vi "test launch & send msg to server.vi"() -> ()   [LabVIEW 2016, in "server.lvlib" / "server.lvclass"]
uses:
  server.lvclass
  C:/Program Files/National Instruments/LabVIEW 2016/vi.lib/ActorFramework/Actor/Actor.lvclass
  <vilib>/ActorFramework/Message Enqueuer/Message Enqueuer.lvclass/Message Enqueuer.ctl
  server Messages/send message to server Msg/send message to server Msg.lvclass/send message to server Msg.ctl
  <vilib>/ActorFramework/Message Enqueuer/Enqueue.vi
  <vilib>/ActorFramework/Stop Msg/Stop Msg.lvclass
  C:/Program Files/National Instruments/LabVIEW 2016/vi.lib/ActorFramework/Message/Message.lvclass
  server Messages/send message to server Msg/send message to server Msg.lvclass
  <vilib>/ActorFramework/Message Priority Queue/Priority Enqueue.vi
  <vilib>/ActorFramework/Message Enqueuer/Message Enqueuer.lvclass
  <vilib>/ActorFramework/Actor/Actor.lvclass
panel:
  in  "event message":string
  in  "send message":bool=TRUE
  in  "stop":bool=TRUE
  # "Launch server"
  # "#这是一个测试server的vi，测试启动、停止server，测试给server发送消息；"
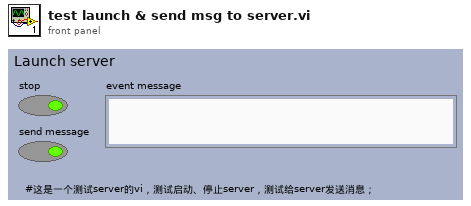
[diagram p1: front panel]
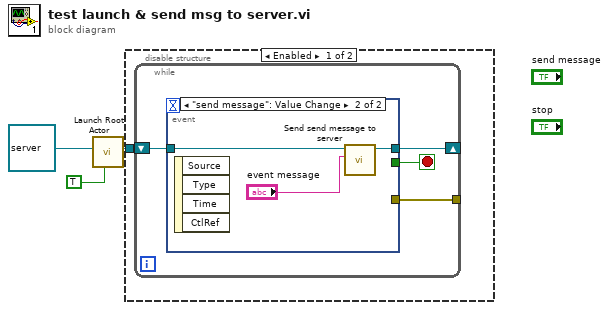
[diagram p0: block diagram]
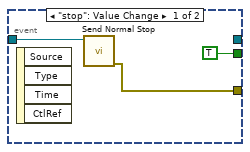
[diagram p2: hidden frame]
diagram:
  n1 = call <vilib>:"Launch Root Actor.vi"("Open Actor Core front panel? (F)"=TRUE, "Actor"=refnum<class "server.lvclass"> refnum ("server.lvlib:server.lvclass")) -> ("Actor's Enqueuer"=w1:refnum<class "Message Enqueuer.lvclass">)  [unwired: 8 in, 1 out]
  n2 = disable-structure shown="Enabled" {
    disable-tunnel: w1 -> [w4 _]
    frame Enabled {
      n3 = while {
        shift-right: [w6] -> _
        shift-left: w4 -> [w8]
        tunnel: [w5] -> _
        stop <- w7 stop-if-true
        n4 = event shown="[1] \"send message\": Value Change" {
          selector: _ -> [_ _]
          dyn-events: _ -> [_ _]
          timeout: _ -> [_ _]
          tunnel: w8 -> [w11 w14]
          tunnel: [TRUE _] -> w7
          tunnel: [_ w13] -> w6
          tunnel: [w9 _] -> w5
          event "stop": Value Change {
            n5 = event-data() -> ()  [unwired: 1 in, 4 out]
            n6 = call <vilib>:"Send Normal Stop.vi"("Message Enqueuer"=w11) -> ("error out"=w9:errorcluster)  [unwired: 10 in]
          }
          event "send message": Value Change {
            n7 = event-data() -> ()  [unwired: 1 in, 4 out]
            n8 = call "Send send message to server.vi"("event message"="event message", "Message Enqueuer"=w14) -> ("Message Enqueuer out"=w13:refnum<class "Message Enqueuer.lvclass">)  [unwired: 8 in, 1 out]
          }
        }
      }
    }
    frame Disabled {
    }
  }
